vi "GetPageProperty.vi"(8 "error in (no error)":errorcluster, 11 "This VI":refnum<vi>) -> (0 "error out":errorcluster, 1 "Settings":variant)   [LabVIEW 2020, in "SLSC-12201 DIO System Explorer.lvlib"]
uses:
  SLSC-12201 DIO System Explorer.lvlib
  Shared/Constants.vi
  Shared/SLSC-12201 DIO Shared.lvlib
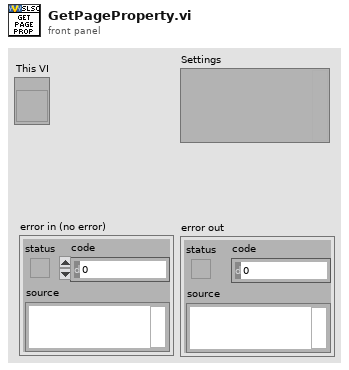
[diagram p1: front panel]
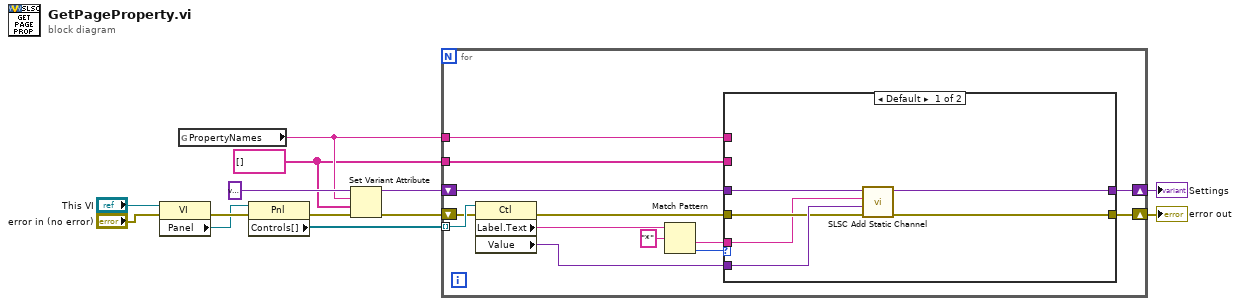
[diagram p0: block diagram]
diagram:
  w1 = string[] []
  n1 = property class="VI"(reference="This VI", error in="error in (no error)") -> (error out=w11:errorcluster, "Panel"=w10:refnum<vi>)  [unwired: 1 out]
  n2 = global read "Constants.vi" "PropertyNames"() -> (w4:string)
  n3 = property class="Pnl"(reference=w10, error in=w11) -> (error out=w3:errorcluster, "Controls[]"=w9:refnum<vi>[])  [unwired: 1 out]
  n4 = Set Variant Attribute(Variant=variant ("variant"), name=w4, value=w1, error in=w3) -> (Variant out=w5:variant, error out=w2:errorcluster)  [unwired: 1 out]
  n5 = for {
    tunnel: w9 -> [w26] mode=indexing
    shift-right: [w20] -> w8
    shift-left: w5 -> [w23]
    shift-right: [w19] -> w7
    shift-left: w2 -> [w25]
    tunnel: w4 -> [w17]
    tunnel: w1 -> [w14]
    n6 = property class="Ctl"(reference=w26, error in=w25) -> (error out=w21:errorcluster, "Label.Text"=w16:string, "Value"=w22:variant)  [unwired: 1 out]
    n7 = Match Pattern(string=w16, regular expression="*") -> (after substring=w18:string, offset past match=w15:i32)  [unwired: 1 in, 2 out]
    n8 = case shown="Default" w15 {
      tunnel: w18 -> [w27 _]
      tunnel: w23 -> [w29 w34]
      tunnel: w22 -> [w32 _]
      tunnel: w21 -> [w28 w33]
      tunnel: [w31 w34] -> w20
      tunnel: [w30 w33] -> w19
      tunnel: w17 -> [_ _]
      tunnel: w14 -> [_ _]
      frame Default {
        n9 = call "SLSC Add Static Channel.vi"("error in (no error)"=w28, "Value"=w32, "Label.Text"=w27, "variant in"=w29) -> ("error out"=w30:errorcluster, "variant out"=w31:variant)  [unwired: 6 in]
      }
      frame -1 {
      }
    }
  }
  "Settings" <- w8
  "error out" <- w7
